vi "Load Categories by Name.vi"(8 "error in (no error)":errorcluster, 10 "String Input":string, 11 "Budgetizer.lvclass":refnum<class "Budgetizer.lvclass">) -> (0 "error out":errorcluster, 2 "Matching Categories":refnum<class "Category.lvclass">[](array[class]), 3 "Budgetizer.lvclass":refnum<class "Budgetizer.lvclass">)   [LabVIEW 2018, in "Budgetizer.lvclass"]
uses:
  Budgetizer.lvclass
  Category/Category.lvclass
  Budgetizer.lvclass/Budgetizer.ctl
  database/Database.lvclass
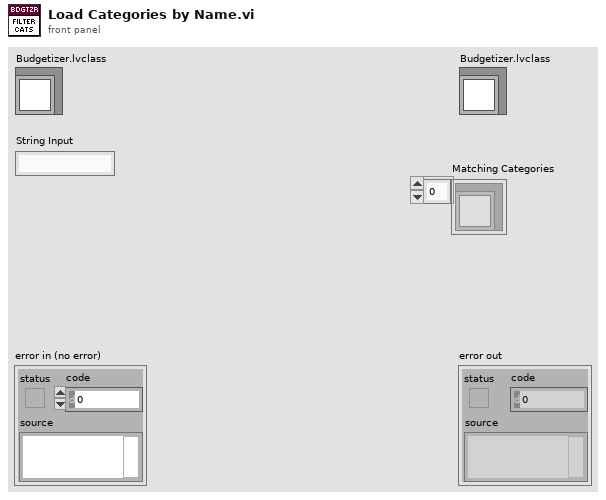
[diagram p1: front panel]
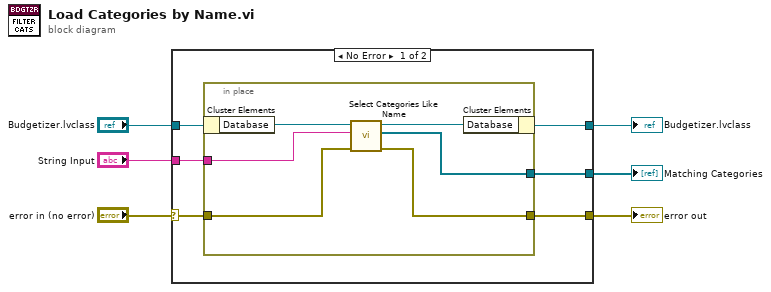
[diagram p0: block diagram]
diagram:
  n1 = case shown="No Error" "error in (no error)" {
    selector: "error in (no error)" -> [w12 w20]
    tunnel: [w11 w20] -> w5
    tunnel: "String Input" -> [w9 _]
    tunnel: [w10 _] -> w3
    tunnel: "Budgetizer.lvclass" -> [w8 w19]
    tunnel: [w7 w19] -> w1
    frame No Error {
      n2 = in-place {
        in-place-border: w12 -> [w16]
        in-place-border: [w14] -> w11
        in-place-border: [w13] -> w10
        in-place-border: w9 -> [w17]
        n3 = in-place-cluster #1(w8) -> ("Database"=w18:refnum<class "Database.lvclass">)
        n4 = call "Select Categories Like Name.vi"("error in (no error)"=w16, "Name filter"=w17, "Database in"=w18) -> ("error out"=w14:errorcluster, "Categories"=w13:refnum<class "Category.lvclass">[], "Database out"=w15:refnum<class "Database.lvclass">)  [unwired: 6 in]
        n5 = in-place-cluster #1("Database"=w15) -> (w7:refnum<class "Budgetizer.lvclass">)
      }
    }
    frame Error {
    }
  }
  "error out" <- w5
  "Matching Categories" <- w3
  "Budgetizer.lvclass" <- w1
